vi "SubVI Frecuencia a Nivel.vi"(11 "Pulp ref":i32) -> (3 "Numeric":dbl)   [LabVIEW 2013]
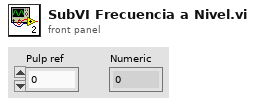
[diagram p1: front panel]
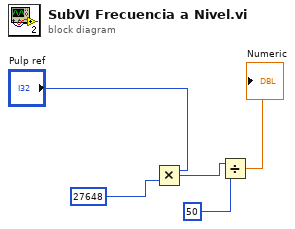
[diagram p0: block diagram]
diagram:
  n1 = Multiply(x="Pulp ref", y=27648) -> (x*y=w3:i32)
  n2 = Divide(x=w3, y=50) -> (x/y=→"Numeric":dbl)
